vi "Query Arb Sequence Capabilities [SEQ] Core.vi"(8 "error in (no error)":errorcluster, 11 "CS++Fgen in":refnum<class "CS++Fgen.lvclass">) -> (0 "error out":errorcluster, 1 "min sequence length":i32, 2 "max number of sequences":i32, 3 "CS++Fgen out":refnum<class "CS++Fgen.lvclass">, 4 "max sequence length":i32, 6 "max loop count":i32)   [LabVIEW 2013, in "CS++Fgen.lvlib" / "CS++Fgen.lvclass"]
doc: "This VI returns the properties of the function generator that are related to creating arbitrary sequences. These properties are the maximum number of sequences, minimum sequence length, maximum sequence length, and maximum loop count.\n\nNotes:\n\n(1) This VI is part of the IviFgenArbSeq [SEQ] extension group."
uses:
  CS++Fgen.lvclass
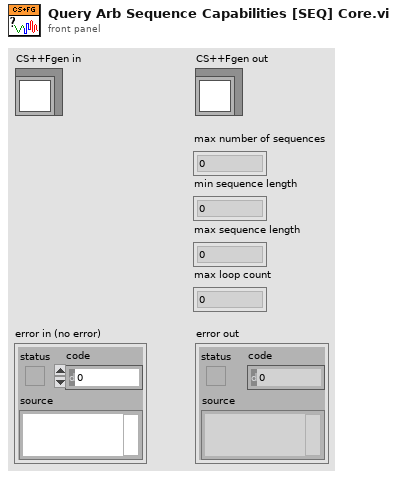
[diagram p1: front panel]
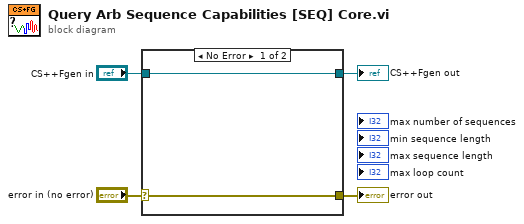
[diagram p0: block diagram]
diagram:
  n1 = case shown="No Error" "error in (no error)" {
    selector: "error in (no error)" -> [w5 w8]
    tunnel: [w5 w8] -> w3
    tunnel: [w6 w7] -> w1
    tunnel: "CS++Fgen in" -> [w6 w7]
    frame No Error {
    }
    frame Error {
    }
  }
  "error out" <- w3
  "CS++Fgen out" <- w1
